vi "ModuleSD.vi"(10 "JQMHStartup.lvclass":refnum<class "RQMHStartup.lvclass">, 11 "JQMHCore in":refnum<class "RQMHModule.lvclass">) -> ()   [LabVIEW 2024, in "RQMHModule.lvclass"]
uses:
  RQMHModule.lvclass
  Startup/RQMHStartup.lvclass
  RQMHModule.lvclass/RQMHModule.ctl
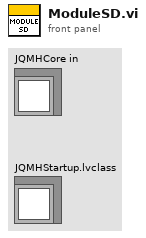
[diagram p1: front panel]
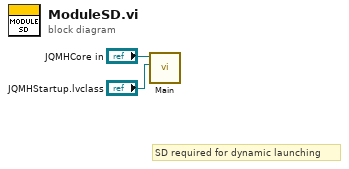
[diagram p0: block diagram]
diagram:
  # "SD required for dynamic launching"
  n1 = call-dynamic "Main.vi"("JQMHStartup.lvclass"="JQMHStartup.lvclass", "JQMHCore in"="JQMHCore in") -> ()  [unwired: 10 in]
